vi "csm_lumikki_instron_stop_poller.vi"   [LabVIEW 2009]
types:
  T1 = cluster{"Device ID":i32, "Device Name":string, "Device Type":i32}[]
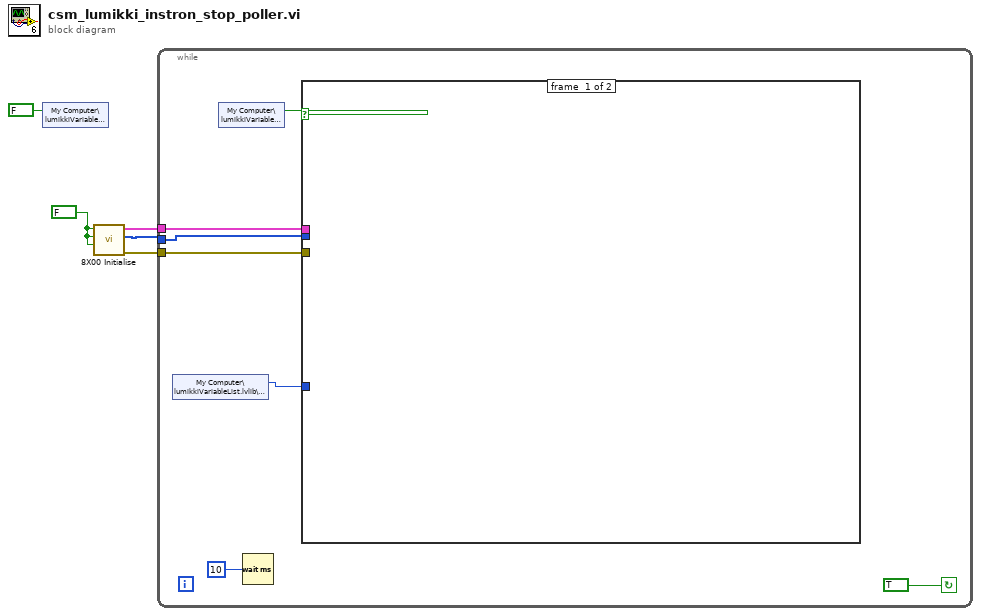
[diagram p0: block diagram]
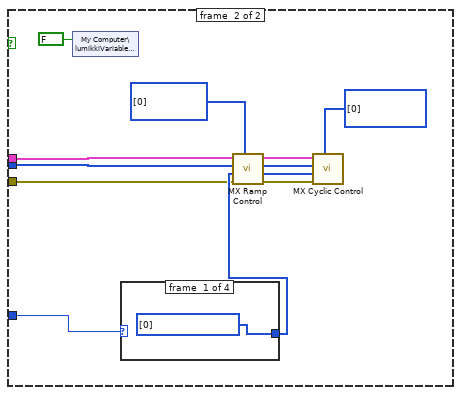
[diagram p2: hidden frame]
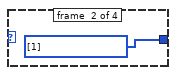
[diagram p3: hidden frame]
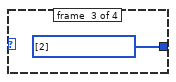
[diagram p4: hidden frame]
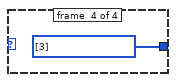
[diagram p5: hidden frame]
diagram:
  w5 = FALSE ("Create Console? (T)")
  n1 = shared-variable "My Computer\\lumikkiVariableList.lvlib\\stop"(FALSE ("stopLogging")) -> ()  [unwired: 1 in, 1 out]
  n2 = call "8X00 Initialise.vi"("Reset?"=w5, "Create DVM? (T)"=w5, "Create Console? (T)"=w5) -> ("error out"=w2:errorcluster, "Axis Selector"=w3:i32[], "Axis Information"=w4:T1)  [unwired: 1 in, 1 out]
  n3 = while {
    tunnel: w4 -> [w11]
    tunnel: w3 -> [w12]
    tunnel: w2 -> [w10]
    stop <- TRUE continue-if-true
    n4 = shared-variable "My Computer\\lumikkiVariableList.lvlib\\channelInt"() -> (w6:i32)  [unwired: 1 in, 1 out]
    n5 = shared-variable "My Computer\\lumikkiVariableList.lvlib\\stop"() -> (w8:bool)  [unwired: 1 in, 1 out]
    n6 = Wait (ms)(milliseconds to wait=u32 10) -> ()  [unwired: 1 out]
    n7 = case shown="True" w8 {
      tunnel: w12 -> [_ w20]
      tunnel: w11 -> [_ w19]
      tunnel: w10 -> [_ w21]
      tunnel: w6 -> [_ w23]
      frame #0 {
      }
      frame #1 {
        w13 = u16[] [0] items=["Stop", "Start or continue", "Hold", "Continue", "Finish current cycle & stop", "Smooth Stop", "Reserved", "Reserved", "Reserved", "Reserved", "Reserved", "Reserved", "Disable", "Enable", "Reserved", "Reserved", "Start/Continue swept waveform", "Dwell at swept frequency"] ("Cyclic Control")
        w14 = u16[] [0] items=["Stop", "Start or continue", "Hold", "Continue", "Return ramp to set level at fixed rate", "Reserved", "Reserved", "Start Random without demand hold", "Start Random with demand hold", "Prepare Random Start without demand hold", "Prepare Random Start with demand hold", "Unslave", "Reserved", "Reserved", "Start Sample Data Playback or Resume", "Prepare for Start of Sample Data", "Reserved", "Reserved", "Resume Playback", "Start an electromechanical frame return"] ("Ramp Control")
        n8 = shared-variable "My Computer\\lumikkiVariableList.lvlib\\stop"(FALSE ("stopLogging")) -> ()  [unwired: 1 in, 1 out]
        n9 = case shown="1, Default" w23 {
          tunnel: [w25 w26 w27 w28] -> w22
          frame #0 {
            w25 = u16[] [0] items=["Channel 1", "Channel 2", "Channel 3", "Channel 4"] ("Choose channel to apply\nthe setpoint")
          }
          frame #1 {
            w26 = u16[] [1] items=["Channel 1", "Channel 2", "Channel 3", "Channel 4"] ("Choose channel to apply\nthe setpoint")
          }
          frame #2 {
            w27 = u16[] [2] items=["Channel 1", "Channel 2", "Channel 3", "Channel 4"] ("Choose channel to apply\nthe setpoint")
          }
          frame #3 {
            w28 = u16[] [3] items=["Channel 1", "Channel 2", "Channel 3", "Channel 4"] ("Choose channel to apply\nthe setpoint")
          }
        }
        n10 = call "MX Ramp Control.vi"("Ramp Control"=w14, "error in (no error)"=w21, "Channels In"=w22, "Axis Selector In"=w20, "Axis Information In"=w19) -> ("error out"=w15:errorcluster, "Channels Out"=w16:u16[], "Axis Selector Out"=w17:i32[], "Axis Information Out"=w18:T1)  [unwired: 2 in]
        n11 = call "MX Cyclic Control.vi"("Cyclic Control"=w13, "error in (no error)"=w15, "Channels"=w16, "Axis Selector"=w17, "Axis Information"=w18) -> ()  [unwired: 2 in, 4 out]
      }
    }
  }
